vi "Initialize.vi"(8 "error in (no error)":errorcluster, 10 "DeviceName":string, 11 "FakePressureController in":refnum<class "MagAnalysis_Online.lvclass">) -> (0 "error out":errorcluster, 1 "new command(s)":string, 2 "DeviceName":string, 3 "FakePressureController out":refnum<class "MagAnalysis_Online.lvclass">)   [LabVIEW 2011, in "MagAnalysis_Online.lvclass"]
uses:
  MagAnalysis_Online.lvclass
  settings_TypDef.ctl
  CamSettings_Typdef.ctl
  CamSettingSUB_TypDEf.ctl
  CamAndObj_TypDEf.ctl
  OnOffTypeDef.ctl
  numericVariable_TypeDef.ctl
  SrewMaster_TYpDef.ctl
  srew_TypDEf.ctl
  ScrewSub_Typdef.ctl
  screwstart.ctl
  dataTypdef.ctl
  IMAQ Image.ctl
  BaseDriver/BaseDriver.lvclass
  MagAnalysis_Online.lvclass/MagAnalysis_Online.ctl
panel:
  in  "data 2":T1
  out "data":T3={"CamSettings"={"Cam 0"={"position"=0.0, "Field of view"=0.0, "start"=0.0, "end"=0.0, "center"=0.0, "Lens"=enum."FL1-f8x08", "Forward"=enum."off", "Spec_Calib_file 2"=path "Y:/100TWdata/ESMCalib/datFwd.txt", "map"=path "Y:/100TWdata/ESMCalib/mapFwd.txt", "y size"=0}, "Cam 1"={"position"=0.0, "Field of view"=0.0, "start"=0.0, "end"=0.0, "center"=0.0, "Lens"=enum."FL1-f8x08", "Forward"=enum."off", "Spec_Calib_file 2"=path "Y:/100TWdata/ESMCalib/datFwd.txt", "map"=path "Y:/100TWdata/ESMCalib/mapFwd.txt", "y size"=0}, "Cam 2"={"position"=0.0, "Field of view"=0.0, "start"=0.0, "end"=0.0, "center"=0.0, "Lens"=enum."FL1-f8x08", "Forward"=enum."off", "Spec_Calib_file 2"=path "Y:/100TWdata/ESMCalib/datFwd.txt", "map"=path "Y:/100TWdata/ESMCalib/mapFwd.txt", "y size"=0}, "Cam 3"={"position"=0.0, "Field of view"=0.0, "start"=0.0, "end"=0.0, "center"=0.0, "Lens"=enum."FL1-f8x08", "Forward"=enum."off", "Spec_Calib_file 2"=path "Y:/100TWdata/ESMCalib/datFwd.txt", "map"=path "Y:/100TWdata/ESMCalib/mapFwd.txt", "y size"=0}}, "timeout"={"Value"=0.0, "Min"=0.0, "Max"=0.0, "StepSize"=0.0, "Tolerance"=0.0, "valueactual"=0.0}, "Screws"={"Cam 0"={"S 0"={"0"=0, "1"=0, "2"=0, "3"=0}, "S 1"={"0"=0, "1"=0, "2"=0, "3"=0}, "S 2"={"0"=0, "1"=0, "2"=0, "3"=0}, "S 3"={"0"=0, "1"=0, "2"=0, "3"=0}, "S 4"={"0"=0, "1"=0, "2"=0, "3"=0}, "S 5"={"0"=0, "1"=0, "2"=0, "3"=0}}, "Cam 1"={"S 0"={"0"=0, "1"=0, "2"=0, "3"=0}, "S 1"={"0"=0, "1"=0, "2"=0, "3"=0}, "S 2"={"0"=0, "1"=0, "2"=0, "3"=0}, "S 3"={"0"=0, "1"=0, "2"=0, "3"=0}, "S 4"={"0"=0, "1"=0, "2"=0, "3"=0}, "S 5"={"0"=0, "1"=0, "2"=0, "3"=0}}, "Cam 2"={"S 0"={"0"=0, "1"=0, "2"=0, "3"=0}, "S 1"={"0"=0, "1"=0, "2"=0, "3"=0}, "S 2"={"0"=0, "1"=0, "2"=0, "3"=0}, "S 3"={"0"=0, "1"=0, "2"=0, "3"=0}, "S 4"={"0"=0, "1"=0, "2"=0, "3"=0}, "S 5"={"0"=0, "1"=0, "2"=0, "3"=0}}, "Cam 3"={"S 0"={"0"=0, "1"=0, "2"=0, "3"=0}, "S 1"={"0"=0, "1"=0, "2"=0, "3"=0}, "S 2"={"0"=0, "1"=0, "2"=0, "3"=0}, "S 3"={"0"=0, "1"=0, "2"=0, "3"=0}, "S 4"={"0"=0, "1"=0, "2"=0, "3"=0}, "S 5"={"0"=0, "1"=0, "2"=0, "3"=0}}}, "number of cam"=0.0, "X size"=0.0, "srewstart"={"Cam 0"=0.0, "Cam 1"=0.0, "Cam 2"=0.0, "Cam 3"=0.0}, "Save"=enum."off", "offset"=0.0, "localsavingpath"=path ""}
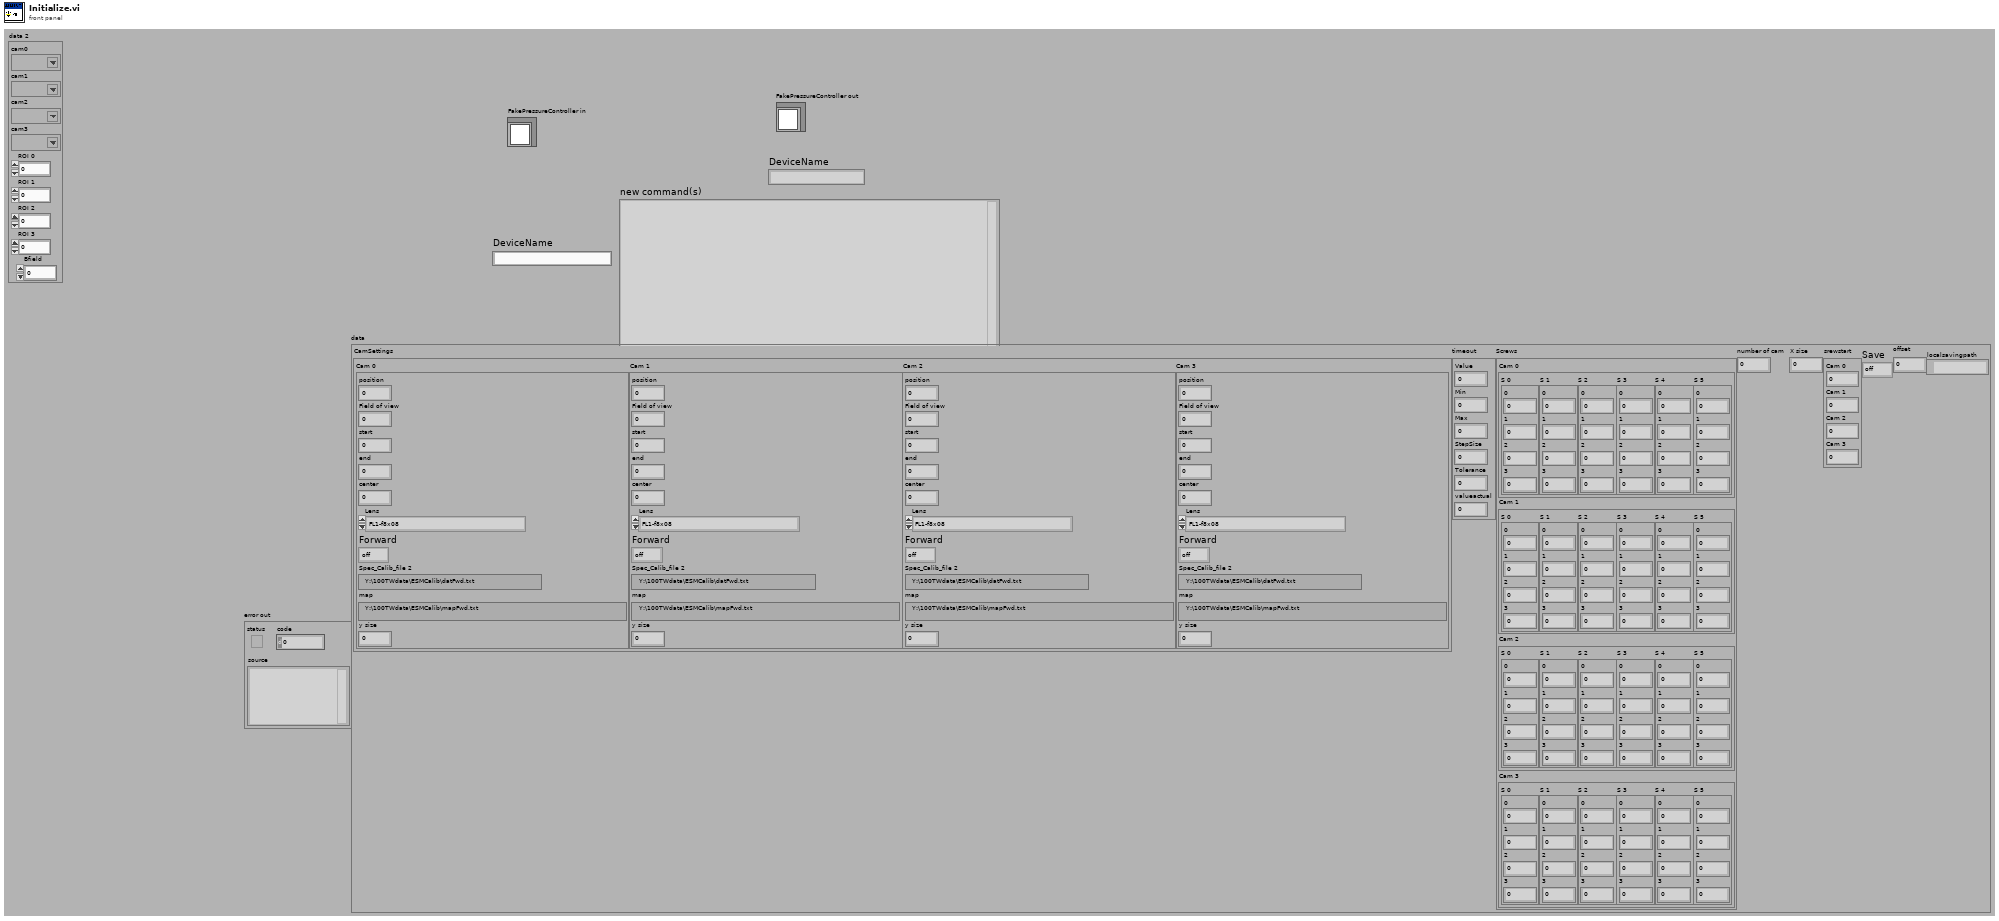
[diagram p1: front panel]
types:
  T1 = typedef "dataTypdef.ctl" = cluster{"cam0":T2, "cam1":T2, "cam2":T2, "cam3":T2, "ROI 0":dbl, "ROI 1":dbl, "ROI 2":dbl, "ROI 3":dbl, "Bfield":dbl}
  T2 = typedef "IMAQ Image.ctl" = refnum<image>
  T3 = typedef "MagAnalysis_Online.lvclass/settings_TypDef.ctl" = cluster{"CamSettings":T4, "timeout":T8, "Screws":T9, "number of cam":dbl, "X size":dbl, "srewstart":T12, "Save":T7, "offset":dbl, "localsavingpath":path}
  T4 = typedef "CamSettings_Typdef.ctl" = cluster{"Cam 0":T5, "Cam 1":T5, "Cam 2":T5, "Cam 3":T5}
  T5 = typedef "CamSettingSUB_TypDEf.ctl" = cluster{"position":dbl, "Field of view":dbl, "start":dbl, "end":dbl, "center":dbl, "Lens":T6, "Forward":T7, "Spec_Calib_file 2":path, "map":path, "y size":i32}
  T6 = typedef "CamAndObj_TypDEf.ctl" = enum16{"FL1-f8x08", "FL1-f8x06", "FL1-f8", "ch300-f50", "FL2G-f8", "FL3M14-f8", "FL3M14-f8x08", "FL3M14-f8x08(2x2)"}
  T7 = typedef "OnOffTypeDef.ctl" = enum16{"off", "on"}
  T8 = typedef "numericVariable_TypeDef.ctl" = cluster{"Value":dbl, "Min":dbl, "Max":dbl, "StepSize":dbl, "Tolerance":dbl, "valueactual":dbl}
  T9 = typedef "SrewMaster_TYpDef.ctl" = cluster{"Cam 0":T10, "Cam 1":T10, "Cam 2":T10, "Cam 3":T10}
  T10 = typedef "srew_TypDEf.ctl" = cluster{"S 0":T11, "S 1":T11, "S 2":T11, "S 3":T11, "S 4":T11, "S 5":T11}
  T11 = typedef "ScrewSub_Typdef.ctl" = cluster{"0":i32, "1":i32, "2":i32, "3":i32}
  T12 = typedef "screwstart.ctl" = cluster{"Cam 0":dbl, "Cam 1":dbl, "Cam 2":dbl, "Cam 3":dbl}
  T13 = typedef "SubscriberCluster_TypDEf.ctl" = cluster{"tcp data event":T14, "Event Registration Refnum":refnum<event-registration>, "data queue":refnum<queue>, "Devices":string[], "Alias":string[], "Variable header":string[], "Devices ALL":string[]}
  T14 = typedef "tcp_new_data_event.ctl" = refnum<user-event>
  T15 = typedef "MagAnalysis_Online.lvclass/analysis_data_typdef.ctl" = cluster{"cam0":T2, "cam1":T2, "cam2":T2, "cam3":T2}
  T16 = typedef "bgImages_tyudef.ctl" = cluster{"cam 0":T2, "cam 1":T2, "cam 2":T2, "cam 3":T2}
  T17 = typedef "calib_Sub_Typdef.ctl" = cluster{"incident ANGLE COMPENSATION":dbl[], "field of view /pixel":dbl, "dp/B [MeV/C/B]":dbl[], "charge compensation":dbl[], "Momentum [MeV/C]":dbl[], "B [T]":dbl, "energyDependence Input":dbl[], "pixel angle (y)":dbl[], "dp [MeV/C/] ":dbl[], "angle 2Dfor spectrumj":dbl[][], "dp [MeV/C] 2D":dbl[][], "charge compensation 2D":dbl[][], "Screen&Camera 2":T18, "ROI info":T19, "Y 2D full angle":dbl[][]}
  T18 = typedef "ScreenCam2_TypDEf.ctl" = cluster{"Screen Orientation":string, "Screen angle":string, "Lens":T6, "Calibration (mm/pix)":dbl}
  T19 = typedef "ROIInfo_TypDef.ctl" = cluster{"npix-X":i32, "npix-Y":i32, "Left [pix]":dbl, "Top [pix]":dbl}
  T20 = cluster{"[0]":T17, "[1]":T17, "[2]":T17, "[3]":T17}
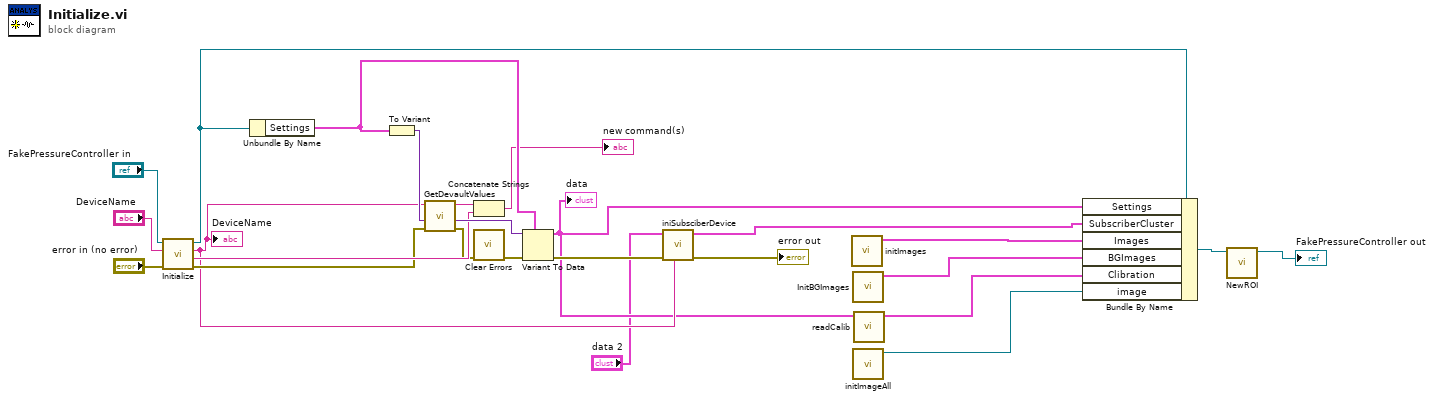
[diagram p0: block diagram]
diagram:
  n1 = call-parent "Initialize.vi"("error in (no error)"="error in (no error)", "DeviceName"="DeviceName", "BaseDriver in"="FakePressureController in") -> ("error out"=w16:errorcluster, "new command(s)"=w18:string, "DeviceName"=w14:string, "BaseDriver out"=w4:refnum<class "MagAnalysis_Online.lvclass">)  [unwired: 5 in]
  "DeviceName" <- w14
  n2 = Unbundle By Name(w4) -> ("Settings"=w19:T3)
  n3 = To Variant(anything=w19) -> (Variant=w20:variant)
  n4 = call "GetDevaultValues.vi"("error in (no error)"=w16, "variant"=w20, "Device Name"=w14) -> ("error out"=w11:errorcluster, "variant out"=w21:variant, "new command(s)"=w22:string)  [unwired: 6 in]
  n5 = Concatenate Strings(w22, w18) -> (→"new command(s)":string)
  n6 = call "Clear Errors.vi"("error in (no error)"=w11) -> ("error out"=w10:errorcluster)  [unwired: 6 in]
  n7 = Variant To Data(error in=w10, type=w19, Variant=w21) -> (data=w5:T3, error out=w15:errorcluster)
  "data" <- w5
  n8 = call "iniSubsciberDevice.vi"("DeviceName"=w14, "error in (no error)"=w15, "variant"="data 2") -> ("error out"=→"error out":errorcluster, "Subscriber cluster"=w13:T13)  [unwired: 7 in]
  n9 = call "initImages.vi"() -> ("output cluster"=w6:T15)  [unwired: 11 in]
  n10 = call "InitBGImages.vi"() -> ("BGImages"=w9:T16)  [unwired: 11 in]
  n11 = call "initImageAll.vi"() -> ("Refnum out"=w8:T2)  [unwired: 11 in]
  n12 = call "readCalib.vi"("Settings"=w5) -> ("Cluster"=w7:T20)  [unwired: 10 in]
  n13 = Bundle By Name(cluster=w4, "Settings"=w5, "SubscriberCluster"=w13, "Images"=w6, "BGImages"=w9, "Clibration"=w7, "image"=w8) -> (w3:refnum<class "MagAnalysis_Online.lvclass">)
  n14 = call "NewROI.vi"("MagAnalysis_Online in"=w3) -> ("MagAnalysis_Online out"=→"FakePressureController out":refnum<class "MagAnalysis_Online.lvclass">)  [unwired: 10 in]
